vi "FPGAController_v4.1.vi"() -> ()   [LabVIEW 2015]
uses:
  <vilib>/Utility/miscctls.llb/LVPointTypeDef.ctl
  <vilib>/FPGAPlugInAG/PXI-7954R/niLvFpga_Open_PXI-7954R.vi
  <userlib>/_OpenG.lib/file/file.llb/Strip Path Extension - Path__ogtk.vi
  <userlib>/_OpenG.lib/comparison/comparison.llb/DBL Changed__ogtk.vi
  <userlib>/_OpenG.lib/comparison/comparison.llb/Boolean Changed__ogtk.vi
  <vilib>/Utility/error.llb/Error Cluster From Error Code.vi
  <vilib>/rvi/errors/niLvFpgaAdjustHostInterfaceError.vi
  <vilib>/addons/database/Connection.llb/Conn Execute.vi
  <vilib>/addons/database/Recordset.llb/Rec Fetch Recordset Data (R).vi
  <vilib>/addons/database/Recordset.llb/Rec Destroy - Connection.vi
  <vilib>/FPGAPlugInAG/PXI-7954R/niLvFpga_Close_PXI-7954R.vi
  <vilib>/rvi/interface/nirviOpenFPGA/nirviOpenFPGA.xnode
  FPGA Bitfiles/correlationwithf_FPGATarget_FPGAcode60214_dpdmgs7o1BA.lvbitx
  <vilib>/rvi/interface/nirviMethod/nirviMethod.xnode
  <vilib>/FPGA/interface/niFpgaViExecutionMode.ctl
  <vilib>/rvi/interface/nirviReadWriteControl/nirviReadWriteControl.xnode
  <vilib>/addons/database/_DB Variant To Data/Database Variant To Data.xnode
  <vilib>/rvi/interface/nirviCloseFPGA/nirviCloseFPGA.xnode
  <vilib>/addons/database/NI_Database_API.lvlib
  NiFpgaLv.dll
panel:
  in  "Tab Control":enum32{"Auto Threshold", "Manual Threshold"}(tab)
  in  "Auto Threshold":bool
  in  "Update All":bool
  in  "Raise Threshold":bool
  in  "Lower Threshold":bool
  in  "Threshold 1":bool
  in  "Threshold 2":bool
  in  "Threshold 3":bool
  in  "Threshold 4":bool
  in  "Threshold 5":bool
  in  "Threshold 6":bool
  in  "Threshold 7":bool
  in  "Update By":i32
  out "Time Betwee Shots":dbl
  out "Del Armed":bool
  out "Update Threshold":bool
  in  "Min. Time\nBetween Shots (s)":dbl
  in  "Rate Limiting":bool
  out "Armed":bool
  in  "Add Delay":bool
  in  "Delay Name":string
  in  "Delay Value":dbl=3.0 min=0.0
  in  "Delay Ring":dbl(ring)=3.15039 items=["Ablation Chamber"=6.45, "LEIL Chamber"=4.318, "Thid Detector"=3.15039, "Custom"=0.0]
  in  "Rearm Trigger":bool
  in  "One Shot Mode":bool
  out "Last Update:":timestamp
  out "Updating FPGA":bool
  out "Sensitivity":dbl
  out "error out":errorcluster
  out "Low Mass Limit":fxp<+,31,17>
  out "High Mass Limit":fxp<+,31,17>
  out "stopping":bool
  out "Peletron (MV)":dbl=2.0
  out "High Mass (kg)":dbl=inf
  out "Low Mass (kg)":dbl
  out "High Charge Limit":i16
  out "Low Charge Limit":i16
  out "High velocity count":i32=210
  out "Low velocity count":i32=21000
  in  "stop":bool
  in  "Peak-Threshold Factor":dbl=2.0
  out "Low Charge Limit (fC)":dbl
  out "High Charge Limit (fC)":dbl=100.0
  out "High Velocity":dbl=100000.0
  out "Low Velocity":dbl=1000.0
  out "Filter 7 Peak":i32=7483
  out "Filter 6 Peak":i32=9863
  out "Filter 5 Peak":i32=13910
  out "Filter 4 Peak":i32=18191
  out "Filter 3 Peak":i32=46254
  out "Filter 2 Peak":i32=120664
  out "Filter 1 Peak":i32=295996
  in  "Filter7 Threshold":i32=-21165
  in  "Filter6 Threshold":i32=-29358
  in  "Filter5 Threshold":i32=-41730
  in  "Filter4 Threshold":i32=-54306
  in  "Filter3 Threshold":i32=-138762
  in  "Filter2 Threshold":i32=-361992
  in  "Filter1 Threshold":i32=-887988
  in  "Zero Peak Values":bool
  in  "Assign Threshold":bool
  in  "Run Mode":bool
  # "Settings"
  # "Dubugging"
  # "Independent Variable"
  # "Low Vel."
  # "High Vel."
  # "Low Q (fC)"
  # "High Q (fC)"
  # "Plate Control While Loop Counter"
  # "Low Mass (kg)"
  # "High Mass (kg)"
  # "Sens. (V/pC)"
  # "Peletron (MV)"
  # "Current Value of Running Average"
  # "Peak Threshold Factor"
  # "Delay Trigger"
  # "Dist. from 2nd Det. (m)"
  # "Name"
  # "Peak Values"
  # "Peak 1"
  # "Peak 2"
  # "Peak 3"
  # "Peak 4"
  # "Peak 5"
  # "Peak 6"
  # "Peak 7"
  # "Thresholds"
  # "Threshold 1"
  # "Threshold 2"
  # "Threshold 3"
  # "Threshold 4"
  # "Threshold 5"
  # "Threshold 6"
  # "Threshold 7"
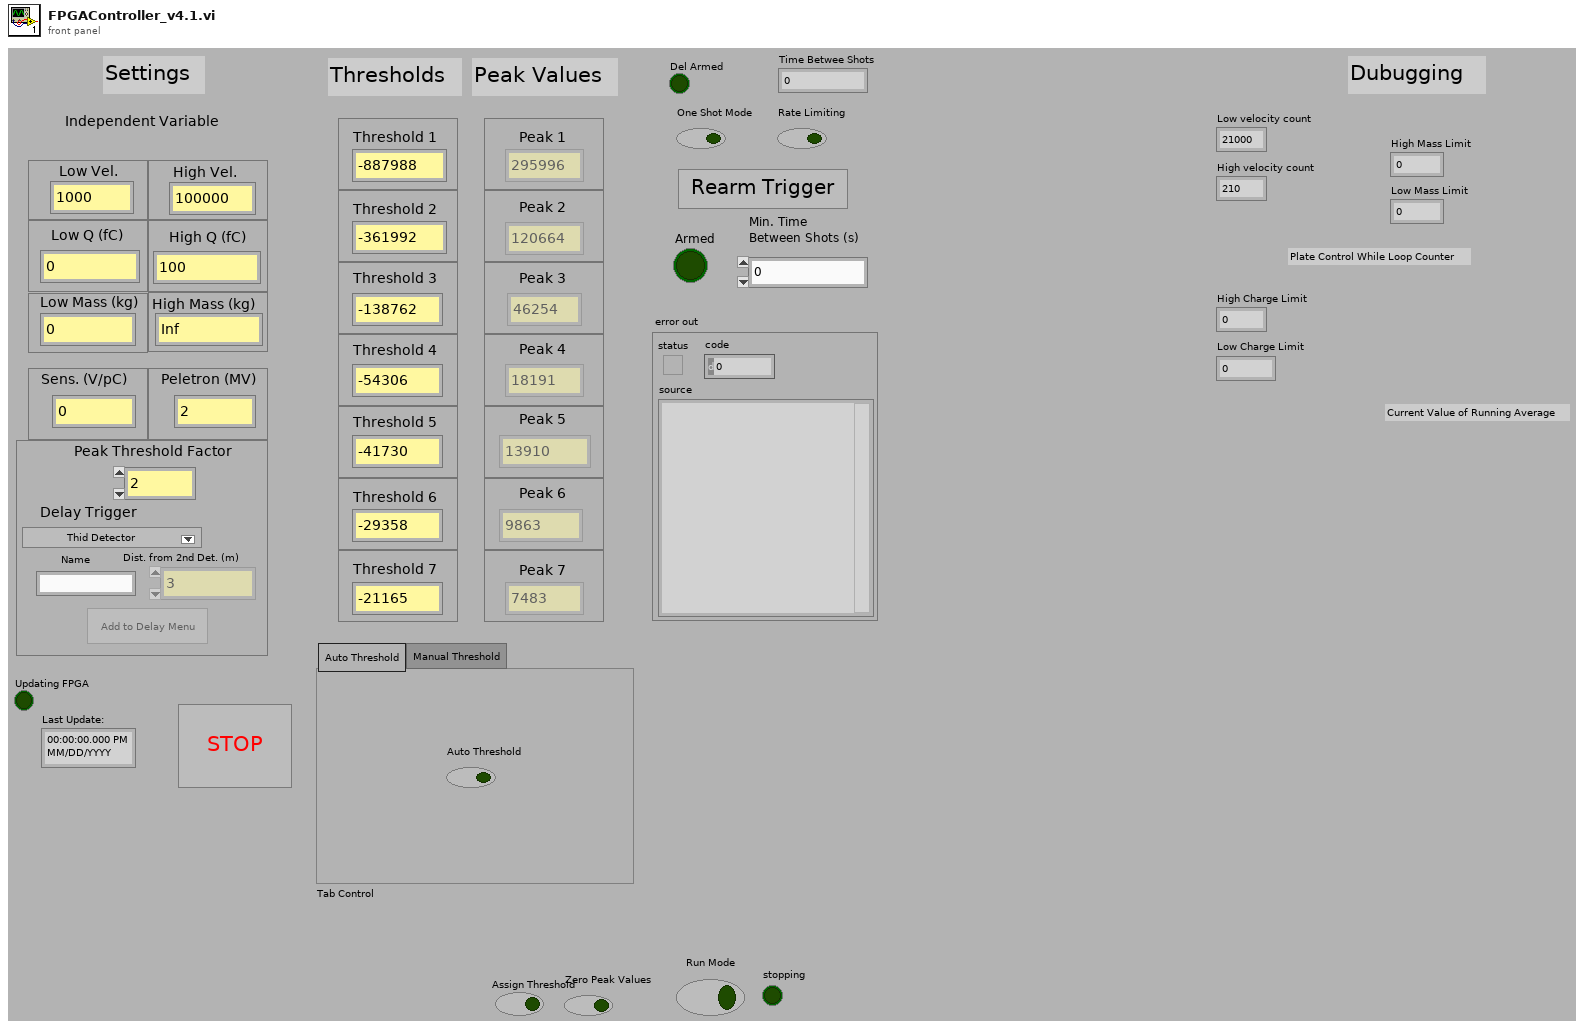
[diagram p1: front panel]
types:
  T1 = typedef "LVPointTypeDef.ctl" = cluster{"Horizontal":i16, "Vertical":i16}
  T2 = enum8{"Enabled", "Disabled", "Disabled and Grayed Out"}
  T3 = typedef "NI_Database_API.lvlib/Conn ObjectReference.ctl" = refnum<k1>
  T4 = cluster{"Filter 1 Peak":i32, "Filter 2 Peak":i32, "Filter 3 Peak":i32, "Filter 4 Peak":i32, "Filter 5 Peak":i32, "Filter 6 Peak":i32, "Filter 7 Peak":i32}
  T5 = typedef "NI_Database_API.lvlib/Rec ObjectReference.ctl" = refnum<k1>
  T6 = typedef "LVStringsAndValuesArrayTypeDef_DBL.ctl" = cluster{"String":string, "Value":dbl}[]
  T7 = cluster{"Numeric":dbl, "Numeric":dbl, "Numeric":dbl, "Numeric":dbl, "Numeric":dbl, "Numeric":dbl, i32, dbl, "Value":dbl, fxp<+,16,7>, bool}
  T8 = cluster{"Low Velocity Count":i32, "High Velocity Count":i32, "Low Charge Limit (ADC ticks)":i16, "High Charge Limit (ADC ticks)":i16, "Low Mass (ADC*cycle^2)":i64, "High Mass (ADC*cycle^2)":i64, "Mult":fxp<+,16,7>, "Mult Use?":bool}
  T9 = cluster{"Filter 1 Detector 3 Correlation":i32, "Filter 2 Detector 3 Correlation":i32, "Filter 3 Detector 3 Correlation":i32, "Filter 4 Detector 3 Correlation":i32, "Filter 5 Detector 3 Correlation":i32, "Filter 6 Detector 3 Correlation":i32, "Filter 7 Detector 3 Correlation":i32}
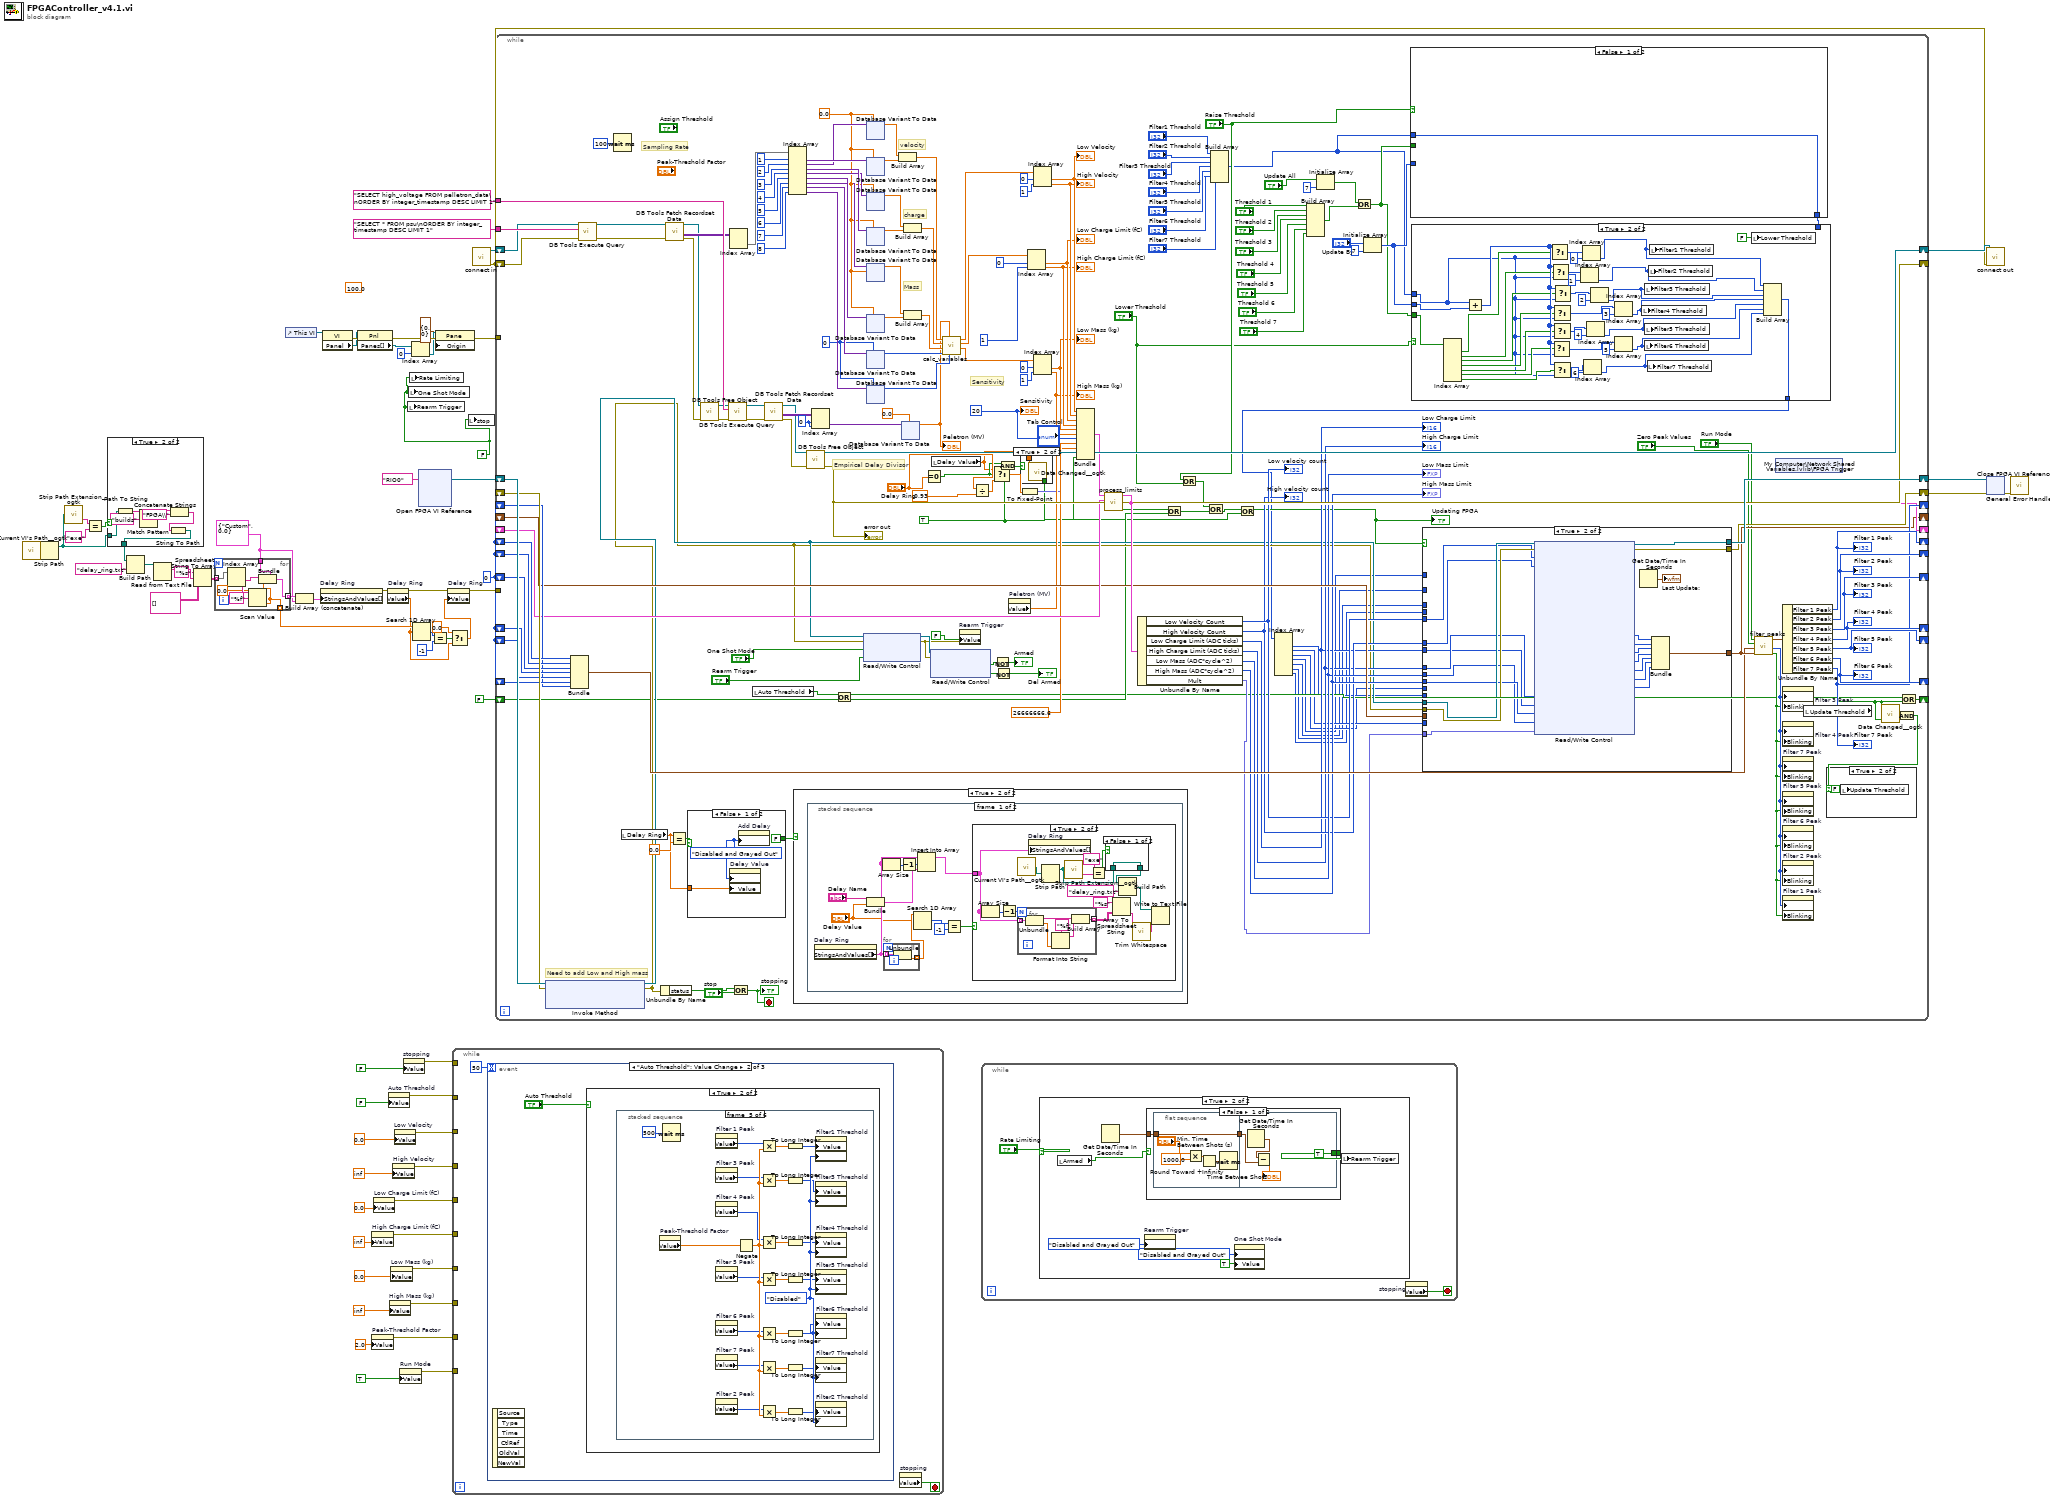
[diagram p0: block diagram]
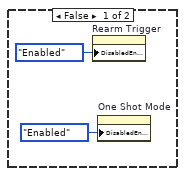
[diagram p3: hidden frame]
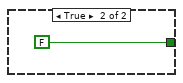
[diagram p4: hidden frame]
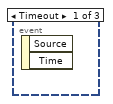
[diagram p5: hidden frame]
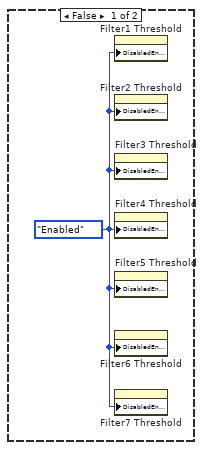
[diagram p6: hidden frame]
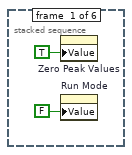
[diagram p7: hidden frame]
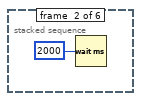
[diagram p8: hidden frame]
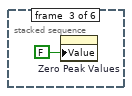
[diagram p9: hidden frame]
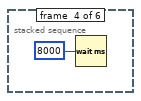
[diagram p10: hidden frame]
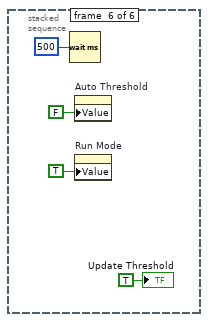
[diagram p11: hidden frame]
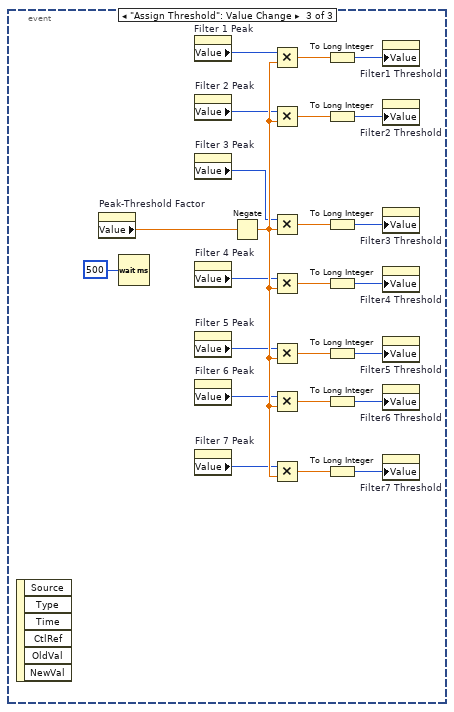
[diagram p12: hidden frame]
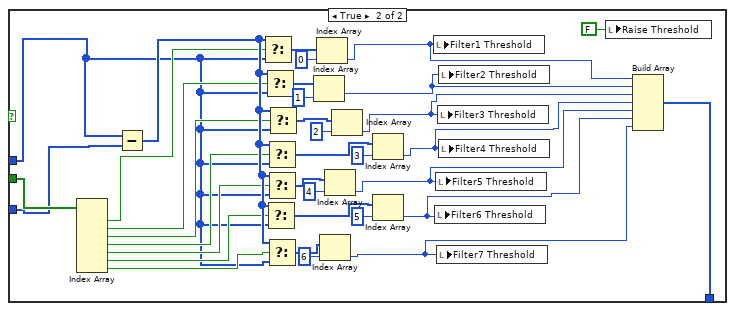
[diagram p14: hidden frame]
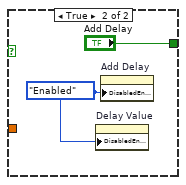
[diagram p17: hidden frame]
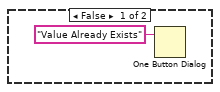
[diagram p19: hidden frame]
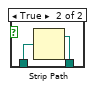
[diagram p20: hidden frame]
diagram:
  (unwired) 100.0 ("Update By")
  w17 = cluster{"String":string, "Value":dbl} {"String"="Custom", "Value"=0.0}
  w27 = FALSE
  w66 = 0
  n1 = call <userlib>:"Current VI's Path__ogtk.vi"() -> ("Current VI's Path (+ Relative)"=w26:path)  [unwired: 1 in]
  n2 = Strip Path(path=w26) -> (stripped path=w12:path)  [unwired: 1 out]
  n3 = call-poly <userlib>:"Strip Path Extension__ogtk.vi"("path"=w12) -> ("extension"=w16:string)  [unwired: 1 out]
  n4 = Equal?(x=w16, y="exe") -> (x = y?=w13:bool)
  n5 = case shown="True" w13 {
    tunnel: w12 -> [w68 w75]
    tunnel: [w68 w69] -> w11
    frame False {
    }
    frame True {
      n6 = Path To String(path=w75) -> (string=w74:string)
      n7 = Match Pattern(string=w74, regular expression="builds") -> (before substring=w72:string)  [unwired: 1 in, 3 out]
      n8 = Concatenate Strings(w72, "FPGA\\" ("string")) -> (w70:string)
      n9 = String To Path(string=w70) -> (path=w69:path)
    }
  }
  n10 = Build Path(base path=w11, name or relative path="delay_ring.txt") -> (appended path=w14:path)
  n11 = Read from Text File(file (use dialog)=w14) -> (text=w24:string)  [unwired: 3 in, 3 out]
  n12 = Spreadsheet String To Array(format string="%s", spreadsheet string=w24, array type (2D Dbl)=string[][] []) -> (array=w21:string[][])  [unwired: 1 in]
  n13 = for {
    tunnel: w21 -> [w83] mode=indexing
    tunnel: w17 -> [w81]
    tunnel: [w77] -> w18 mode=indexing
    tunnel: [w76] -> w10 mode=indexing
    n14 = Index Array(array=w83) -> (element #1=w82:string, element #2=w80:string)  [unwired: 2 in]
    n15 = Scan Value(string=w80, format string="%f", default (0 dbl)=0.0) -> (value=w76:dbl)  [unwired: 1 out]
    n16 = Bundle(cluster=w81, "String"=w82, "Value"=w76) -> (w77:cluster{"String":string, "Value":dbl})
  }
  n17 = control-ref of="This VI"() -> (w38:refnum<vi>)
  n18 = Build Array (concatenate)(w18, w17) -> (w20:cluster{"String":string, "Value":dbl}[])
  n19 = property on="Delay Ring" class="Ring (strict)"("StringsAndValues[]"=w20) -> (error out=w19:errorcluster)  [unwired: 2 in, 1 out]
  n20 = property class="VI"(reference=w38) -> (error out=w37:errorcluster, "Panel"=w36:refnum<vi>)  [unwired: 1 in, 1 out]
  n21 = property class="Pnl"(reference=w36, error in=w37) -> (error out=w35:errorcluster, "Panes[]"=w34:refnum<vi>[])  [unwired: 1 out]
  n22 = property on="High Charge Limit (fC)" class="DigNum (strict)"("Value"=inf ("High Charge Limit (fC)")) -> (error out=w53:errorcluster)  [unwired: 2 in, 1 out]
  n23 = property on="Peak-Threshold Factor" class="DigNum (strict)"("Value"=2.0 ("Peak-Threshold Factor")) -> (error out=w47:errorcluster)  [unwired: 2 in, 1 out]
  n24 = property on="Low Charge Limit (fC)" class="DigNum (strict)"("Value"=0.0 ("Low Charge Limit (fC)")) -> (error out=w55:errorcluster)  [unwired: 2 in, 1 out]
  n25 = property on="Delay Ring" class="Ring (strict)"(error in=w19) -> (error out=w9:errorcluster, "Value"=w3:dbl)  [unwired: 1 in, 1 out]
  n26 = property on="Auto Threshold" class="Bool (strict)"("Value"=FALSE ("Auto Threshold")) -> (error out=w61:errorcluster)  [unwired: 2 in, 1 out]
  n27 = property on="High Mass (kg)" class="DigNum (strict)"("Value"=inf ("High Mass (kg)")) -> (error out=w49:errorcluster)  [unwired: 2 in, 1 out]
  n28 = property on="Low Mass (kg)" class="DigNum (strict)"("Value"=0.0 ("Low Mass (kg)")) -> (error out=w51:errorcluster)  [unwired: 2 in, 1 out]
  n29 = property on="High Velocity" class="DigNum (strict)"("Value"=inf ("High Velocity")) -> (error out=w57:errorcluster)  [unwired: 2 in, 1 out]
  n30 = property on="Low Velocity" class="DigNum (strict)"("Value"=0.0 ("Low Velocity")) -> (error out=w59:errorcluster)  [unwired: 2 in, 1 out]
  n31 = property on="Run Mode" class="Bool (strict)"("Value"=TRUE ("Run Mode")) -> (error out=w45:errorcluster)  [unwired: 2 in, 1 out]
  n32 = property on="stopping" class="Bool (strict)"("Value"=FALSE ("stopping")) -> (error out=w63:errorcluster)  [unwired: 2 in, 1 out]
  n33 = local write "Rearm Trigger"(w27) -> ()
  n34 = local write "One Shot Mode"(w27) -> ()
  n35 = local write "Rate Limiting"(w27) -> ()
  n36 = Index Array(array=w34, index=0) -> (element=w32:refnum<vi>)
  n37 = Search 1D Array(1D array=w10, element=w3) -> (index of element=w7:i32)  [unwired: 1 in]
  n38 = xnode "Open FPGA VI Reference"("resource name"=tag "RIO0") -> ("FPGA VI Reference Out"=w29:refnum<k20>)  [unwired: 1 in, 1 out]
  n39 = Equal?(x=w7, y=-1) -> (x = y?=w5:bool)
  n40 = property class="Pane"(reference=w32, error in=w35, "Origin"=T1 {"Horizontal"=0, "Vertical"=0}) -> (error out=w30:errorcluster)  [unwired: 1 out]
  n41 = Select(t=0.0, s=w5, f=w3) -> (s? t:f=w4:dbl)
  n42 = property on="Delay Ring" class="Ring (strict)"(error in=w9, "Value"=w4) -> (error out=w8:errorcluster)  [unwired: 1 in, 1 out]
  n43 = while {
    tunnel: w63 -> [_]
    tunnel: w61 -> [_]
    tunnel: w59 -> [_]
    tunnel: w57 -> [_]
    tunnel: w55 -> [_]
    tunnel: w53 -> [_]
    tunnel: w51 -> [_]
    tunnel: w49 -> [_]
    tunnel: w47 -> [_]
    tunnel: w45 -> [_]
    stop <- w85 stop-if-true
    n44 = event shown="[1] \"Auto Threshold\": Value Change" {
      selector: _ -> [_ _ _]
      dyn-events: _ -> [_ _ _]
      timeout: 50 -> [_ _ _]
      event Timeout {
        n45 = event-data() -> ()  [unwired: 1 in, 2 out]
      }
      event "Auto Threshold": Value Change {
        n46 = event-data() -> ()  [unwired: 1 in, 6 out]
        n47 = case shown="True" "Auto Threshold" {
          frame False {
            w87 = T2."Enabled" ("Disabled")
            n48 = property on="Filter1 Threshold" class="DigNum (strict)"("DisabledEnum"=w87) -> ()  [unwired: 2 in, 2 out]
            n49 = property on="Filter2 Threshold" class="DigNum (strict)"("DisabledEnum"=w87) -> ()  [unwired: 2 in, 2 out]
            n50 = property on="Filter3 Threshold" class="DigNum (strict)"("DisabledEnum"=w87) -> ()  [unwired: 2 in, 2 out]
            n51 = property on="Filter4 Threshold" class="DigNum (strict)"("DisabledEnum"=w87) -> ()  [unwired: 2 in, 2 out]
            n52 = property on="Filter5 Threshold" class="DigNum (strict)"("DisabledEnum"=w87) -> ()  [unwired: 2 in, 2 out]
            n53 = property on="Filter6 Threshold" class="DigNum (strict)"("DisabledEnum"=w87) -> ()  [unwired: 2 in, 2 out]
            n54 = property on="Filter7 Threshold" class="DigNum (strict)"("DisabledEnum"=w87) -> ()  [unwired: 2 in, 2 out]
          }
          frame True {
            n55 = stacked-sequence {
              frame #0 {
                n56 = property on="Zero Peak Values" class="Bool (strict)"("Value"=TRUE ("Zero Peak Values")) -> ()  [unwired: 2 in, 2 out]
                n57 = property on="Run Mode" class="Bool (strict)"("Value"=FALSE ("Run Mode")) -> ()  [unwired: 2 in, 2 out]
              }
              frame #1 {
                n58 = Wait (ms)(milliseconds to wait=u32 2000) -> ()  [unwired: 1 out]
              }
              frame #2 {
                n59 = property on="Zero Peak Values" class="Bool (strict)"("Value"=FALSE ("Zero Peak Values")) -> ()  [unwired: 2 in, 2 out]
              }
              frame #3 {
                n60 = Wait (ms)(milliseconds to wait=u32 8000) -> ()  [unwired: 1 out]
              }
              frame #4 {
                w117 = T2."Disabled" ("Disabled")
                n61 = property on="Peak-Threshold Factor" class="DigNum (strict)"() -> ("Value"=w102:dbl)  [unwired: 2 in, 2 out]
                n62 = Wait (ms)(milliseconds to wait=u32 500) -> ()  [unwired: 1 out]
                n63 = property on="Filter 1 Peak" class="DigNum (strict)"() -> ("Value"=w100:i32)  [unwired: 2 in, 2 out]
                n64 = property on="Filter 3 Peak" class="DigNum (strict)"() -> ("Value"=w98:i32)  [unwired: 2 in, 2 out]
                n65 = property on="Filter 4 Peak" class="DigNum (strict)"() -> ("Value"=w97:i32)  [unwired: 2 in, 2 out]
                n66 = property on="Filter 5 Peak" class="DigNum (strict)"() -> ("Value"=w96:i32)  [unwired: 2 in, 2 out]
                n67 = property on="Filter 6 Peak" class="DigNum (strict)"() -> ("Value"=w95:i32)  [unwired: 2 in, 2 out]
                n68 = property on="Filter 7 Peak" class="DigNum (strict)"() -> ("Value"=w94:i32)  [unwired: 2 in, 2 out]
                n69 = property on="Filter 2 Peak" class="DigNum (strict)"() -> ("Value"=w99:i32)  [unwired: 2 in, 2 out]
                n70 = Negate(x=w102) -> (-x=w101:dbl)
                n71 = Multiply(x=w100, y=w101) -> (x*y=w116:dbl)
                n72 = Multiply(x=w98, y=w101) -> (x*y=w112:dbl)
                n73 = Multiply(x=w97, y=w101) -> (x*y=w110:dbl)
                n74 = Multiply(x=w96, y=w101) -> (x*y=w108:dbl)
                n75 = Multiply(x=w95, y=w101) -> (x*y=w106:dbl)
                n76 = Multiply(x=w94, y=w101) -> (x*y=w104:dbl)
                n77 = Multiply(x=w99, y=w101) -> (x*y=w114:dbl)
                n78 = To Long Integer(number=w116) -> (32bit integer=w115:i32)
                n79 = To Long Integer(number=w112) -> (32bit integer=w111:i32)
                n80 = To Long Integer(number=w110) -> (32bit integer=w109:i32)
                n81 = To Long Integer(number=w108) -> (32bit integer=w107:i32)
                n82 = To Long Integer(number=w106) -> (32bit integer=w105:i32)
                n83 = To Long Integer(number=w104) -> (32bit integer=w103:i32)
                n84 = To Long Integer(number=w114) -> (32bit integer=w113:i32)
                n85 = property on="Filter1 Threshold" class="DigNum (strict)"("Value"=w115, "DisabledEnum"=w117) -> ()  [unwired: 2 in, 2 out]
                n86 = property on="Filter3 Threshold" class="DigNum (strict)"("Value"=w111, "DisabledEnum"=w117) -> ()  [unwired: 2 in, 2 out]
                n87 = property on="Filter4 Threshold" class="DigNum (strict)"("Value"=w109, "DisabledEnum"=w117) -> ()  [unwired: 2 in, 2 out]
                n88 = property on="Filter5 Threshold" class="DigNum (strict)"("Value"=w107, "DisabledEnum"=w117) -> ()  [unwired: 2 in, 2 out]
                n89 = property on="Filter6 Threshold" class="DigNum (strict)"("Value"=w105, "DisabledEnum"=w117) -> ()  [unwired: 2 in, 2 out]
                n90 = property on="Filter7 Threshold" class="DigNum (strict)"("Value"=w103, "DisabledEnum"=w117) -> ()  [unwired: 2 in, 2 out]
                n91 = property on="Filter2 Threshold" class="DigNum (strict)"("Value"=w113, "DisabledEnum"=w117) -> ()  [unwired: 2 in, 2 out]
              }
              frame #5 {
                n92 = Wait (ms)(milliseconds to wait=u32 500) -> ()  [unwired: 1 out]
                n93 = property on="Auto Threshold" class="Bool (strict)"("Value"=FALSE ("Auto Threshold")) -> ()  [unwired: 2 in, 2 out]
                n94 = property on="Run Mode" class="Bool (strict)"("Value"=TRUE ("Run Mode")) -> ()  [unwired: 2 in, 2 out]
                "Update Threshold" <- TRUE ("Update Threshold")
              }
            }
          }
        }
      }
      event "Assign Threshold": Value Change {
        n95 = event-data() -> ()  [unwired: 1 in, 6 out]
        n96 = property on="Peak-Threshold Factor" class="DigNum (strict)"() -> ("Value"=w136:dbl)  [unwired: 2 in, 2 out]
        n97 = Wait (ms)(milliseconds to wait=u32 500) -> ()  [unwired: 1 out]
        n98 = property on="Filter 1 Peak" class="DigNum (strict)"() -> ("Value"=w135:i32)  [unwired: 2 in, 2 out]
        n99 = property on="Filter 2 Peak" class="DigNum (strict)"() -> ("Value"=w134:i32)  [unwired: 2 in, 2 out]
        n100 = property on="Filter 3 Peak" class="DigNum (strict)"() -> ("Value"=w133:i32)  [unwired: 2 in, 2 out]
        n101 = property on="Filter 4 Peak" class="DigNum (strict)"() -> ("Value"=w132:i32)  [unwired: 2 in, 2 out]
        n102 = property on="Filter 5 Peak" class="DigNum (strict)"() -> ("Value"=w131:i32)  [unwired: 2 in, 2 out]
        n103 = property on="Filter 6 Peak" class="DigNum (strict)"() -> ("Value"=w130:i32)  [unwired: 2 in, 2 out]
        n104 = property on="Filter 7 Peak" class="DigNum (strict)"() -> ("Value"=w129:i32)  [unwired: 2 in, 2 out]
        n105 = Negate(x=w136) -> (-x=w138:dbl)
        n106 = Multiply(x=w135, y=w138) -> (x*y=w145:dbl)
        n107 = Multiply(x=w134, y=w138) -> (x*y=w143:dbl)
        n108 = Multiply(x=w133, y=w138) -> (x*y=w142:dbl)
        n109 = Multiply(x=w132, y=w138) -> (x*y=w141:dbl)
        n110 = Multiply(x=w131, y=w138) -> (x*y=w140:dbl)
        n111 = Multiply(x=w130, y=w138) -> (x*y=w139:dbl)
        n112 = Multiply(x=w129, y=w138) -> (x*y=w144:dbl)
        n113 = To Long Integer(number=w145) -> (32bit integer=w128:i32)
        n114 = To Long Integer(number=w143) -> (32bit integer=w127:i32)
        n115 = To Long Integer(number=w142) -> (32bit integer=w126:i32)
        n116 = To Long Integer(number=w141) -> (32bit integer=w125:i32)
        n117 = To Long Integer(number=w140) -> (32bit integer=w124:i32)
        n118 = To Long Integer(number=w139) -> (32bit integer=w123:i32)
        n119 = To Long Integer(number=w144) -> (32bit integer=w122:i32)
        n120 = property on="Filter1 Threshold" class="DigNum (strict)"("Value"=w128) -> ()  [unwired: 2 in, 2 out]
        n121 = property on="Filter2 Threshold" class="DigNum (strict)"("Value"=w127) -> ()  [unwired: 2 in, 2 out]
        n122 = property on="Filter3 Threshold" class="DigNum (strict)"("Value"=w126) -> ()  [unwired: 2 in, 2 out]
        n123 = property on="Filter4 Threshold" class="DigNum (strict)"("Value"=w125) -> ()  [unwired: 2 in, 2 out]
        n124 = property on="Filter5 Threshold" class="DigNum (strict)"("Value"=w124) -> ()  [unwired: 2 in, 2 out]
        n125 = property on="Filter6 Threshold" class="DigNum (strict)"("Value"=w123) -> ()  [unwired: 2 in, 2 out]
        n126 = property on="Filter7 Threshold" class="DigNum (strict)"("Value"=w122) -> ()  [unwired: 2 in, 2 out]
      }
    }
    n127 = property on="stopping" class="Bool (strict)"() -> ("Value"=w85:bool)  [unwired: 2 in, 2 out]
  }
  n128 = local write "stop"(w27) -> ()
  n129 = call "connect in.vi"() -> ("error out"=w39:errorcluster, "Database Connection"=w40:T3)  [unwired: 7 in, 1 out]
  n130 = while {
    shift-right: [w322] -> w65
    shift-left: w29 -> [w326]
    shift-right: [w321] -> w64
    shift-left: _ -> [w325]
    shift-right: [w317] -> _
    shift-left: w66 -> [w310]
    shift-right: [w316] -> _
    shift-left: w66 -> [w309]
    shift-right: [w315] -> _
    shift-left: w66 -> [w308]
    shift-right: [w314] -> _
    shift-left: w66 -> [w307]
    shift-right: [w313] -> _
    shift-left: w66 -> [w306]
    shift-right: [w319] -> _
    shift-left: w66 -> [w312]
    shift-right: [w318] -> _
    shift-left: w66 -> [w311]
    tunnel: "SELECT * FROM psu\nORDER BY integer_timestamp DESC LIMIT 1" ("SQL query") -> [w305]
    tunnel: "SELECT high_voltage FROM pelletron_data\nORDER BY integer_timestamp DESC LIMIT 1" ("SQL query") -> [w304]
    shift-right: [w300] -> w41
    shift-left: w40 -> [w303]
    shift-right: [w301] -> _
    shift-left: w39 -> [w302]
    shift-right: [w299] -> _
    shift-left: _ -> [w298]
    shift-right: [w296] -> _
    shift-left: _ -> [w297]
    tunnel: w30 -> [_]
    tunnel: w8 -> [_]
    shift-right: [w200] -> _
    shift-left: FALSE -> [w203]
    stop <- w320 stop-if-true
    w168 = TRUE
    w252 = 0 ("index (row)")
    w260 = i8 0
    w261 = 0.0
    w226 = 20
    # "charge"
    # "Empirical Delay Divisor"
    # "Mass"
    # "velocity"
    # "Sensitivity"
    # "Sampling Rate"
    # "Need to add Low and High mass"
    n131 = xnode "Invoke Method"("FPGA VI Reference In"=w326, "error in"=w325) -> ("FPGA VI Reference Out"=w220:refnum<k20>, "error out"=w219:errorcluster)  [unwired: 1 out]
    n132 = Bundle("Filter 1 Peak"=w312, "Filter 2 Peak"=w311, "Filter 3 Peak"=w310, "Filter 4 Peak"=w309, "Filter 5 Peak"=w308, "Filter 6 Peak"=w307, "Filter 7 Peak"=w306) -> (w292:T4)  [unwired: 1 in]
    n133 = call-poly <vilib>:"DB Tools Execute Query.vi"("error in (no error)"=w302, "SQL query"=w305, "connection reference"=w303) -> ("error out"=w280:errorcluster, "recordset reference"=w281:T5)  [unwired: 5 in]
    n134 = Wait (ms)(milliseconds to wait=u32 100) -> ()  [unwired: 1 out]
    n135 = local read "Delay Ring"() -> (w204:dbl)
    n136 = Unbundle By Name(w219) -> ("status"=w324:bool)
    n137 = call-poly <vilib>:"DB Tools Fetch Recordset Data.vi"("error in (no error)"=w280, "recordset reference"=w281) -> ("error out"=w258:errorcluster, "recordset data"=w271:variant[][], "recordset reference out"=w259:T5)  [unwired: 3 in]
    n138 = Equal?(x=w204, y=0.0) -> (x = y?=w205:bool)
    n139 = case shown="False" w205 {
      tunnel: [FALSE ("Add Delay") "Add Delay"] -> w223
      tunnel: w204 -> [w402 _]
      frame False {
        w403 = T2."Disabled and Grayed Out" ("Disabled")
        n140 = property on="Delay Value" class="DigNum (strict)"("DisabledEnum"=w403, "Value"=w402) -> ()  [unwired: 2 in, 2 out]
        n141 = property on="Add Delay" class="Bool (strict)"("DisabledEnum"=w403) -> ()  [unwired: 2 in, 2 out]
      }
      frame True {
        w404 = T2."Enabled" ("Disabled")
        n142 = property on="Delay Value" class="DigNum (strict)"("DisabledEnum"=w404) -> ()  [unwired: 2 in, 2 out]
        n143 = property on="Add Delay" class="Bool (strict)"("DisabledEnum"=w404) -> ()  [unwired: 2 in, 2 out]
      }
    }
    n144 = call-poly <vilib>:"DB Tools Free Object.vi"("error in (no error)"=w258, "recordset reference"=w259) -> ("error out"=w256:errorcluster, "connection reference"=w257:T3)  [unwired: 8 in]
    n145 = call-poly <vilib>:"DB Tools Execute Query.vi"("error in (no error)"=w256, "SQL query"=w304, "connection reference"=w257) -> ("error out"=w254:errorcluster, "recordset reference"=w255:T5)  [unwired: 5 in]
    n146 = Index Array(array=w271) -> (element=w270:variant[])  [unwired: 2 in]
    n147 = Or(x=w324, y="stop") -> (x .or. y?=w320:bool)
    "stopping" <- w320
    n148 = local read "Auto Threshold"() -> (w201:bool)
    n149 = call-poly <vilib>:"DB Tools Fetch Recordset Data.vi"("error in (no error)"=w254, "recordset reference"=w255) -> ("error out"=w227:errorcluster, "recordset data"=w253:variant[][], "recordset reference out"=w228:T5)  [unwired: 3 in]
    n150 = Index Array(array=w270, index #1=1 ("index"), index #2=2 ("index"), index #3=3 ("index"), index #4=4 ("index"), index #5=5 ("index"), index #6=6 ("index"), index #7=7 ("index"), index #8=8 ("index")) -> (element #1=w269:variant, element #2=w268:variant, element #3=w267:variant, element #4=w266:variant, element #5=w265:variant, element #6=w264:variant, element #7=w263:variant, element #8=w262:variant)
    n151 = case shown="True" w223 {
      frame False {
      }
      frame True {
        n152 = stacked-sequence {
          frame #0 {
            n153 = property on="Delay Ring" class="Ring (strict)"() -> ("StringsAndValues[]"=w408:T6)  [unwired: 2 in, 2 out]
            n154 = Bundle("Delay Name"="Delay Name", "Delay Value"="Delay Value") -> (w413:cluster{"Delay Name":string, "Delay Value":dbl})  [unwired: 1 in]
            n155 = Array Size(array=w408) -> (size(s)=w411:i32)
            n156 = for {
              tunnel: w408 -> [w418] mode=indexing
              tunnel: [w417] -> w407 mode=indexing
              n157 = Unbundle(w418) -> ("Value"=w417:dbl)  [unwired: 1 out]
            }
            n158 = Decrement(x=w411) -> (x-1=w410:i32)
            n159 = Search 1D Array(1D array=w407, element="Delay Value") -> (index of element=w415:i32)  [unwired: 1 in]
            n160 = Insert Into Array(array=w408, index=w410, new element=w413) -> (w412:T6)
            n161 = Equal?(x=w415, y=-1) -> (x = y?=w409:bool)
            n162 = case shown="True" w409 {
              tunnel: w412 -> [_ w427]
              frame False {
                n163 = One Button Dialog(message="Value Already Exists") -> ()  [unwired: 1 in, 1 out]
              }
              frame True {
                n164 = Array Size(array=w427) -> (size(s)=w429:i32)
                n165 = Decrement(x=w429) -> (x-1=w428:i32)
                n166 = call <userlib>:"Current VI's Path__ogtk.vi"() -> ("Current VI's Path (+ Relative)"=w433:path)  [unwired: 1 in]
                n167 = for {
                  N: w428 -> [_]
                  tunnel: w427 -> [w443] mode=indexing
                  tunnel: [w438] -> w430 mode=indexing
                  n168 = Unbundle(w443) -> ("String"=w439:string, "Value"=w442:dbl)
                  n169 = Format Into String(format string="%f", w442) -> (resulting string=w440:string)  [unwired: 2 in, 1 out]
                  n170 = Build Array(w439, w440) -> (w438:string[])
                }
                n171 = property on="Delay Ring" class="Ring (strict)"("StringsAndValues[]"=w427) -> ()  [unwired: 2 in, 2 out]
                n172 = Strip Path(path=w433) -> (stripped path=w421:path)  [unwired: 1 out]
                n173 = call-poly <userlib>:"Strip Path Extension__ogtk.vi"("path"=w421) -> ("extension"=w424:string)  [unwired: 1 out]
                n174 = Equal?(x="exe", y=w424) -> (x = y?=w422:bool)
                n175 = case shown="False" w422 {
                  tunnel: w421 -> [w435 w437]
                  tunnel: [w435 w436] -> w420
                  frame False {
                  }
                  frame True {
                    n176 = Strip Path(path=w437) -> (stripped path=w436:path)  [unwired: 1 out]
                  }
                }
                n177 = Array To Spreadsheet String(array=w430, 3:"%s" ("format string")) -> (spreadsheet string=w426:string)  [unwired: 1 in]
                n178 = Build Path(base path=w420, name or relative path="delay_ring.txt") -> (appended path=w431:path)
                n179 = call <vilib>:"Trim Whitespace.vi"("string"=w426) -> ("trimmed string"=w425:string)  [unwired: 1 in]
                n180 = Write to Text File(file (use dialog)=w431, text=w425) -> ()  [unwired: 2 in, 3 out]
              }
            }
          }
          frame #1 {
            n181 = property on="Add Delay" class="Bool (strict)"("Value"=FALSE ("Add Delay")) -> ()  [unwired: 2 in, 2 out]
          }
        }
      }
    }
    n182 = call-poly <vilib>:"DB Tools Free Object.vi"("error in (no error)"=w227, "recordset reference"=w228) -> ("error out"=w301:errorcluster, "connection reference"=w300:T3)  [unwired: 8 in]
    "error out" <- w301
    n183 = Index Array(array=w253, index (row)=w252, index (col)=w252) -> (element=w251:variant)
    n184 = Or(x=w201, y=w203) -> (x .or. y?=w202:bool)
    n185 = xnode "Read/Write Control"("FPGA VI Reference In"=w220, "error in"=w219, "One Shot"="One Shot Mode", "Reset One Shot"="Rearm Trigger") -> ("FPGA VI Reference Out"=w213:refnum<k20>, "error out"=w212:errorcluster)
    n186 = xnode "Database Variant To Data"("database variant"=w268, "type"=w261) -> ("data"=w179:dbl)  [unwired: 1 in, 1 out]
    n187 = xnode "Database Variant To Data"("database variant"=w269, "type"=w261) -> ("data"=w180:dbl)  [unwired: 1 in, 1 out]
    n188 = xnode "Database Variant To Data"("database variant"=w266, "type"=w261) -> ("data"=w178:dbl)  [unwired: 1 in, 1 out]
    n189 = xnode "Database Variant To Data"("database variant"=w267, "type"=w261) -> ("data"=w177:dbl)  [unwired: 1 in, 1 out]
    n190 = xnode "Database Variant To Data"("database variant"=w264, "type"=w261) -> ("data"=w176:dbl)  [unwired: 1 in, 1 out]
    n191 = xnode "Database Variant To Data"("database variant"=w265, "type"=w261) -> ("data"=w175:dbl)  [unwired: 1 in, 1 out]
    n192 = xnode "Database Variant To Data"("database variant"=w263, "type"=w260) -> ("data"=w245:i8)  [unwired: 1 in, 1 out]
    n193 = xnode "Database Variant To Data"("database variant"=w262, "type"=w260) -> ("data"=w244:i8)  [unwired: 1 in, 1 out]
    n194 = Build Array(w179, w180) -> (w248:dbl[])
    n195 = xnode "Database Variant To Data"("database variant"=w251, "type"=0.0) -> ("data"=w174:dbl)  [unwired: 1 in, 1 out]
    "Peletron (MV)" <- w174
    n196 = Build Array(w178, w177) -> (w247:dbl[])
    n197 = Build Array(w176, w175) -> (w246:dbl[])
    n198 = Equal To 0?(x="Delay Ring") -> (x = 0?=w173:bool)
    n199 = xnode "Read/Write Control"("FPGA VI Reference In"=w213, "error in"=w212) -> ("Not Armed?"=w211:bool, "Del Not Armed?"=w167:bool)  [unwired: 2 out]
    n200 = local read "Delay Value"() -> (w172:dbl)
    n201 = call "calc_variables.vi"("var2"=w244, "Peletron"=w174, "var1"=w245, "Mass"=w246, "Charge"=w247, "Velocity"=w248) -> ("Mass out"=w237:dbl[], "Charge out"=w240:dbl[], "Velocity out"=w243:dbl[])  [unwired: 3 in]
    n202 = property on="Rearm Trigger" class="Bool (strict)"(error in=w212, "Value"=FALSE ("Rearm Trigger")) -> ()  [unwired: 1 in, 2 out]
    n203 = Divide(x="Delay Ring", y=0.93) -> (x/y=w209:dbl)
    n204 = Select(t=w172, s=w173, f=w209) -> (s? t:f=w208:dbl)
    n205 = Not(x=w211) -> (.not. x?=→"Armed":bool)
    n206 = Not(x=w167) -> (.not. x?=→"Del Armed":bool)
    n207 = And(x=w173, y=w168) -> (x .and. y?=w169:bool)
    n208 = property on="Peletron (MV)" class="DigNum (strict)"() -> ("Value"=w249:dbl)  [unwired: 2 in, 2 out]
    n209 = case shown="True" w169 {
      selector: w169 -> [w397 _]
      tunnel: w172 -> [_ w399]
      tunnel: [w397 w398] -> w170
      frame False {
      }
      frame True {
        n210 = call-poly <userlib>:"Data Changed__ogtk.vi"("DBL"=w399) -> ("Changed"=w398:bool)
      }
    }
    n211 = To Fixed-Point(number=w208) -> (fixed-point=w222:fxp<+,16,7>)  [unwired: 1 in]
    n212 = Index Array(array=w240, index #1=0 ("index"), index #2=1 ("index")) -> (element #1=w232:dbl, element #2=w231:dbl)
    "High Charge Limit (fC)" <- w231
    "Low Charge Limit (fC)" <- w232
    n213 = Index Array(array=w243, index #1=0 ("index"), index #2=1 ("index")) -> (element #1=w234:dbl, element #2=w233:dbl)
    "High Velocity" <- w233
    "Low Velocity" <- w234
    n214 = Index Array(array=w237, index #1=0 ("index"), index #2=1 ("index")) -> (element #1=w230:dbl, element #2=w229:dbl)
    "Low Mass (kg)" <- w230
    "High Mass (kg)" <- w229
    n215 = Bundle("Numeric"=w234, "Numeric"=w233, "Numeric"=w232, "Numeric"=w231, "Numeric"=w230, "Numeric"=w229, w226, 26666666.6, "Value"=w249, w222, w168) -> (w291:T7)  [unwired: 1 in]
    n216 = call "process_limits.vi"("old output cluster"=w298, "Input cluster"=w291) -> ("Update FPGA"=w225:bool, "output cluster"=w299:T8)  [unwired: 8 in]
    n217 = Unbundle By Name(w299) -> ("Low Velocity Count"=w287:i32, "High Velocity Count"=w286:i32, "Low Charge Limit (ADC ticks)"=w284:i16, "High Charge Limit (ADC ticks)"=w285:i16, "Low Mass (ADC*cycle^2)"=w289:i64, "High Mass (ADC*cycle^2)"=w290:i64, "Mult"=w221:fxp<+,16,7>)
    "Low velocity count" <- w287
    "High velocity count" <- w286
    "High Charge Limit" <- w285
    "Low Charge Limit" <- w284
    "High Mass Limit" <- w290
    "Low Mass Limit" <- w289
    n218 = Or(x=w225, y=w202) -> (x .or. y?=w207:bool)
    n219 = Or(x="Raise Threshold", y="Lower Threshold") -> (x .or. y?=w181:bool)
    n220 = Or(x=w181, y=w207) -> (x .or. y?=w182:bool)
    n221 = Build Array("Filter1 Threshold", "Filter2 Threshold", "Filter3 Threshold", "Filter4 Threshold", "Filter5 Threshold", "Filter6 Threshold", "Filter7 Threshold") -> (w148:i32[])
    n222 = Or(x=w182, y=w170) -> (x .or. y?=w171:bool)
    "Updating FPGA" <- w171
    n223 = Build Array("Threshold 1", "Threshold 2", "Threshold 3", "Threshold 4", "Threshold 5", "Threshold 6", "Threshold 7") -> (w155:bool[])
    n224 = Initialize Array("Update All", 7 ("dimension size")) -> (w156:bool[])
    n225 = Or(x=w156, y=w155) -> (x .or. y?=w149:bool[])
    n226 = Initialize Array("Update By", 7 ("dimension size")) -> (w150:i32[])
    n227 = case shown="False" "Raise Threshold" {
      tunnel: w148 -> [w362 w373]
      tunnel: w149 -> [_ w374]
      tunnel: w150 -> [_ w372]
      tunnel: [w362 w363] -> w147
      frame False {
      }
      frame True {
        n228 = Index Array(array=w374) -> (element #1=w395:bool, element #2=w394:bool, element #3=w393:bool, element #4=w392:bool, element #5=w391:bool, element #6=w390:bool, element #7=w389:bool)  [unwired: 7 in]
        n229 = Subtract(x=w373, y=w372) -> (x-y=w396:i32[])
        n230 = Select(t=w396, s=w395, f=w373) -> (s? t:f=w388:i32[])
        n231 = Select(t=w396, s=w394, f=w373) -> (s? t:f=w384:i32[])
        n232 = Select(t=w396, s=w390, f=w373) -> (s? t:f=w377:i32[])
        n233 = Select(t=w396, s=w392, f=w373) -> (s? t:f=w381:i32[])
        n234 = Select(t=w396, s=w391, f=w373) -> (s? t:f=w379:i32[])
        n235 = Select(t=w396, s=w389, f=w373) -> (s? t:f=w375:i32[])
        n236 = Select(t=w396, s=w393, f=w373) -> (s? t:f=w383:i32[])
        n237 = Index Array(array=w384, index=1) -> (element=w369:i32)
        n238 = Index Array(array=w388, index=0) -> (element=w370:i32)
        n239 = Index Array(array=w375, index=6) -> (element=w364:i32)
        n240 = Index Array(array=w379, index=4) -> (element=w366:i32)
        n241 = Index Array(array=w383, index=2) -> (element=w368:i32)
        n242 = Index Array(array=w381, index=3) -> (element=w367:i32)
        n243 = Index Array(array=w377, index=5) -> (element=w365:i32)
        n244 = local write "Filter1 Threshold"(w370) -> ()
        n245 = local write "Filter6 Threshold"(w365) -> ()
        n246 = local write "Filter5 Threshold"(w366) -> ()
        n247 = local write "Filter7 Threshold"(w364) -> ()
        n248 = local write "Filter3 Threshold"(w368) -> ()
        n249 = local write "Filter2 Threshold"(w369) -> ()
        n250 = local write "Filter4 Threshold"(w367) -> ()
        n251 = local write "Raise Threshold"(FALSE ("Raise Threshold")) -> ()
        n252 = Build Array(w370, w369, w368, w367, w366, w365, w364) -> (w363:i32[])
      }
    }
    n253 = case shown="True" "Lower Threshold" {
      tunnel: w148 -> [_ w351]
      tunnel: w150 -> [_ w361]
      tunnel: w149 -> [_ w360]
      tunnel: [w327 w328] -> w146
      tunnel: w147 -> [w327 _]
      frame False {
      }
      frame True {
        n254 = Index Array(array=w360) -> (element #1=w358:bool, element #2=w357:bool, element #3=w356:bool, element #4=w355:bool, element #5=w354:bool, element #6=w353:bool, element #7=w352:bool)  [unwired: 7 in]
        n255 = Add(x=w351, y=w361) -> (x+y=w359:i32[])
        n256 = Select(t=w359, s=w358, f=w351) -> (s? t:f=w350:i32[])
        n257 = Select(t=w359, s=w357, f=w351) -> (s? t:f=w346:i32[])
        n258 = Select(t=w359, s=w353, f=w351) -> (s? t:f=w339:i32[])
        n259 = Select(t=w359, s=w355, f=w351) -> (s? t:f=w343:i32[])
        n260 = Select(t=w359, s=w354, f=w351) -> (s? t:f=w341:i32[])
        n261 = Select(t=w359, s=w352, f=w351) -> (s? t:f=w337:i32[])
        n262 = Select(t=w359, s=w356, f=w351) -> (s? t:f=w345:i32[])
        n263 = Index Array(array=w346, index=1) -> (element=w334:i32)
        n264 = Index Array(array=w350, index=0) -> (element=w335:i32)
        n265 = Index Array(array=w337, index=6) -> (element=w329:i32)
        n266 = Index Array(array=w341, index=4) -> (element=w331:i32)
        n267 = Index Array(array=w345, index=2) -> (element=w333:i32)
        n268 = Index Array(array=w343, index=3) -> (element=w332:i32)
        n269 = Index Array(array=w339, index=5) -> (element=w330:i32)
        n270 = local write "Filter4 Threshold"(w332) -> ()
        n271 = local write "Filter6 Threshold"(w330) -> ()
        n272 = local write "Filter3 Threshold"(w333) -> ()
        n273 = local write "Filter5 Threshold"(w331) -> ()
        n274 = local write "Filter7 Threshold"(w329) -> ()
        n275 = local write "Filter2 Threshold"(w334) -> ()
        n276 = local write "Filter1 Threshold"(w335) -> ()
        n277 = local write "Lower Threshold"(FALSE ("Lower Threshold")) -> ()
        n278 = Build Array(w335, w334, w333, w332, w331, w330, w329) -> (w328:i32[])
      }
    }
    n279 = Index Array(array=w146) -> (element #1=w195:i32, element #2=w193:i32, element #3=w191:i32, element #4=w189:i32, element #5=w187:i32, element #6=w185:i32, element #7=w183:i32)  [unwired: 7 in]
    n280 = case shown="True" w171 {
      tunnel: w220 -> [w446 w467]
      tunnel: w219 -> [w447 w466]
      tunnel: [w446 w465] -> w322
      tunnel: [w447 w464] -> w321
      tunnel: w195 -> [_ _]
      tunnel: w193 -> [_ _]
      tunnel: w191 -> [_ _]
      tunnel: w189 -> [_ _]
      tunnel: w187 -> [_ _]
      tunnel: w185 -> [_ _]
      tunnel: w183 -> [_ _]
      tunnel: [w445 w450] -> w296
      tunnel: w290 -> [_ w456]
      tunnel: w289 -> [_ w455]
      tunnel: w287 -> [_ w454]
      tunnel: w286 -> [_ w453]
      tunnel: w285 -> [_ w452]
      tunnel: w284 -> [_ w451]
      tunnel: w297 -> [w445 _]
      tunnel: w221 -> [_ w448]
      frame False {
      }
      frame True {
        n281 = xnode "Read/Write Control"("FPGA VI Reference In"=w467, "error in"=w466, "Low Velocity Count"=w454, "High Velocity Count"=w453, "High Charge Limit"=w452, "Low Charge Limit"=w451, "High Mass Limit"=w456, "Low Mass Limit"=w455, "Mult1"=w448) -> ("FPGA VI Reference Out"=w465:refnum<k20>, "error out"=w464:errorcluster, "Filter 1 Detector 3 Correlation"=w463:i32, "Filter 2 Detector 3 Correlation"=w462:i32, "Filter 3 Detector 3 Correlation"=w461:i32, "Filter 4 Detector 3 Correlation"=w460:i32, "Filter 5 Detector 3 Correlation"=w459:i32, "Filter 6 Detector 3 Correlation"=w458:i32, "Filter 7 Detector 3 Correlation"=w457:i32)  [unwired: 7 in]
        n282 = Get Date/Time In Seconds() -> (seconds since 1Jan1904=→"Last Update:":timestamp)
        n283 = Bundle("Filter 1 Detector 3 Correlation"=w463, "Filter 2 Detector 3 Correlation"=w462, "Filter 3 Detector 3 Correlation"=w461, "Filter 4 Detector 3 Correlation"=w460, "Filter 5 Detector 3 Correlation"=w459, "Filter 6 Detector 3 Correlation"=w458, "Filter 7 Detector 3 Correlation"=w457) -> (w450:T9)  [unwired: 1 in]
      }
    }
    n284 = call "filter_peaks.vi"("Correlation cluster"=w296, "Filter peak cluster"=w292, "Zero out"="Zero Peak Values", "Run Mode"="Run Mode") -> ("Blinking"=w283:bool, "status"=w288:T2, "Filter peak output"=w293:T4)  [unwired: 5 in]
    n285 = shared-variable "My Computer\\Network Shared Variables.lvlib\\FPGA Trigger"() -> ()  [unwired: 1 in, 2 out]
    n286 = Unbundle By Name(w293) -> ("Filter 1 Peak"=w319:i32, "Filter 2 Peak"=w318:i32, "Filter 3 Peak"=w317:i32, "Filter 4 Peak"=w316:i32, "Filter 5 Peak"=w315:i32, "Filter 6 Peak"=w314:i32, "Filter 7 Peak"=w313:i32)
    "Filter 1 Peak" <- w319
    "Filter 2 Peak" <- w318
    "Filter 3 Peak" <- w317
    "Filter 4 Peak" <- w316
    "Filter 5 Peak" <- w315
    "Filter 6 Peak" <- w314
    "Filter 7 Peak" <- w313
    n287 = property on="Filter 3 Peak" class="DigNum (strict)"("DisabledEnum"=w288, "Blinking"=w283) -> ()  [unwired: 2 in, 2 out]
    n288 = property on="Filter 4 Peak" class="DigNum (strict)"("DisabledEnum"=w288, "Blinking"=w283) -> ()  [unwired: 2 in, 2 out]
    n289 = property on="Filter 7 Peak" class="DigNum (strict)"("DisabledEnum"=w288, "Blinking"=w283) -> ()  [unwired: 2 in, 2 out]
    n290 = property on="Filter 5 Peak" class="DigNum (strict)"("DisabledEnum"=w288, "Blinking"=w283) -> ()  [unwired: 2 in, 2 out]
    n291 = property on="Filter 6 Peak" class="DigNum (strict)"("DisabledEnum"=w288, "Blinking"=w283) -> ()  [unwired: 2 in, 2 out]
    n292 = property on="Filter 2 Peak" class="DigNum (strict)"("DisabledEnum"=w288, "Blinking"=w283) -> ()  [unwired: 2 in, 2 out]
    n293 = property on="Filter 1 Peak" class="DigNum (strict)"("DisabledEnum"=w288, "Blinking"=w283) -> ()  [unwired: 2 in, 2 out]
    n294 = local read "Update Threshold"() -> (w198:bool)
    n295 = call-poly <userlib>:"Data Changed__ogtk.vi"("Boolean"=w198) -> ("Changed"=w199:bool)
    n296 = And(x=w199, y=w198) -> (x .and. y?=w197:bool)
    n297 = case shown="True" w197 {
      frame False {
      }
      frame True {
        n298 = local write "Update Threshold"(FALSE ("Update Threshold")) -> ()
      }
    }
    n299 = Or(x=w201, y=w198) -> (x .or. y?=w200:bool)
    "Sensitivity" <- w226
  }
  n300 = while {
    stop <- w757 stop-if-true
    n301 = case shown="True" "Rate Limiting" {
      frame False {
        n302 = property on="Rearm Trigger" class="Bool (strict)"("DisabledEnum"=T2."Enabled" ("Disabled")) -> ()  [unwired: 2 in, 2 out]
        n303 = property on="One Shot Mode" class="Bool (strict)"("DisabledEnum"=T2."Enabled" ("Disabled")) -> ()  [unwired: 2 in, 2 out]
      }
      frame True {
        n304 = local read "Armed"() -> (w761:bool)
        n305 = Get Date/Time In Seconds() -> (seconds since 1Jan1904=w760:timestamp)
        n306 = property on="Rearm Trigger" class="Bool (strict)"("DisabledEnum"=T2."Disabled and Grayed Out" ("Disabled")) -> ()  [unwired: 2 in, 2 out]
        n307 = case shown="False" w761 {
          tunnel: [w768 FALSE] -> w765
          tunnel: w760 -> [w767 _]
          frame False {
            n308 = flat-sequence {
              tunnel: w767 -> [w769]
              tunnel: [w769] -> w766
              tunnel: [TRUE] -> w768
              tunnel: w766 -> [w775]
              frame #0 {
                n309 = Multiply(x="Min. Time\nBetween Shots (s)", y=1000.0) -> (x*y=w772:dbl)
                n310 = Round Toward +Infinity(x=w772) -> (ceil(x): smallest int >= x=w770:dbl)
                n311 = Wait (ms)(milliseconds to wait=w770) -> ()  [unwired: 1 out]
              }
              frame #1 {
                n312 = Get Date/Time In Seconds() -> (seconds since 1Jan1904=w776:timestamp)
                n313 = Subtract(x=w776, y=w775) -> (x-y=→"Time Betwee Shots":dbl)
              }
            }
          }
          frame True {
          }
        }
        n314 = property on="One Shot Mode" class="Bool (strict)"("DisabledEnum"=T2."Disabled and Grayed Out" ("Disabled"), "Value"=TRUE ("One Shot Mode")) -> ()  [unwired: 2 in, 2 out]
        n315 = local write "Rearm Trigger"(w765) -> ()
      }
    }
    n316 = property on="stopping" class="Bool (strict)"() -> ("Value"=w757:bool)  [unwired: 2 in, 2 out]
  }
  n317 = call "connect out.vi"("error in (no error)"=w39, "connection reference"=w41) -> ()  [unwired: 9 in, 1 out]
  n318 = xnode "Close FPGA VI Reference"("FPGA VI Reference In"=w65, "error in"=w64) -> ("error out"=w67:errorcluster)
  n319 = call <vilib>:"General Error Handler.vi"("error in (no error)"=w67) -> ()  [unwired: 10 in, 5 out]
